vi "DSF.Shared.Configuration.Transfer.Initialize.vi"(7 "direction":T1, 8 "error in (no error)":errorcluster, 10 "Transfer Configuration cluster":T2, 11 "Transfer Configuration in":refnum<class "VeriStand DSF.Transfer.Configuration.lvclass">) -> (0 "error out":errorcluster, 3 "Transfer Configuration out":refnum<class "VeriStand DSF.Transfer.Configuration.lvclass">)   [LabVIEW 2017, in "Data Sharing Framework Engine.lvlib" / "VeriStand DSF.Transfer.Configuration.lvclass"]
uses:
  VeriStand DSF.Transfer.Configuration.lvclass
  DSF Core/Built/PharLap x86/Engine/c/DSF.Engine.lvlibp/DSF Configuration API/1.0.0/Public/Controls/DSF Engine Transfer Configuration.ctl
  DSF Core/Built/PharLap x86/Engine/c/DSF.Engine.lvlibp/DSF Configuration API/1.0.0/Public/Controls/DSF Byte Order.ctl
  DSF Core/Built/PharLap x86/Engine/c/DSF.Engine.lvlibp/DSF Configuration API/1.0.0/Public/Controls/DSF Engine Channel Configuration.ctl
  DSF Core/Built/PharLap x86/Engine/c/DSF.Engine.lvlibp/DSF Configuration API/1.0.0/Public/Controls/DSF Data Type.ctl
  DSF Core/Built/PharLap x86/Engine/c/DSF.Engine.lvlibp/DSF Configuration API/1.0.0/Public/Controls/DSF Settings Info.ctl
  DSF Core/Built/PharLap x86/Engine/c/DSF.Engine.lvlibp/DSF Configuration API/1.0.0/Public/Controls/DSF Direction.ctl
  VeriStand DSF.Transfer.Configuration.lvclass/VeriStand DSF.Transfer.Configuration.ctl
  <vilib>/NI Veristand/Custom Device API/Custom Device Channel Type.ctl
  <vilib>/NI Veristand/Custom Device API/Data Access Type.ctl
  DSF Core/Built/PharLap x86/Engine/c/DSF.Engine.lvlibp/Shared/Classes/Transfer/DSF.Shared.Configuration.Transfer.lvclass
  <vilib>/NI Veristand/Custom Device API/Custom Device API.lvlib
  DSF Core/Built/PharLap x86/Engine/c/DSF.Engine.lvlibp/DSF Configuration API/1.0.0/DSF Configuration API.lvlib
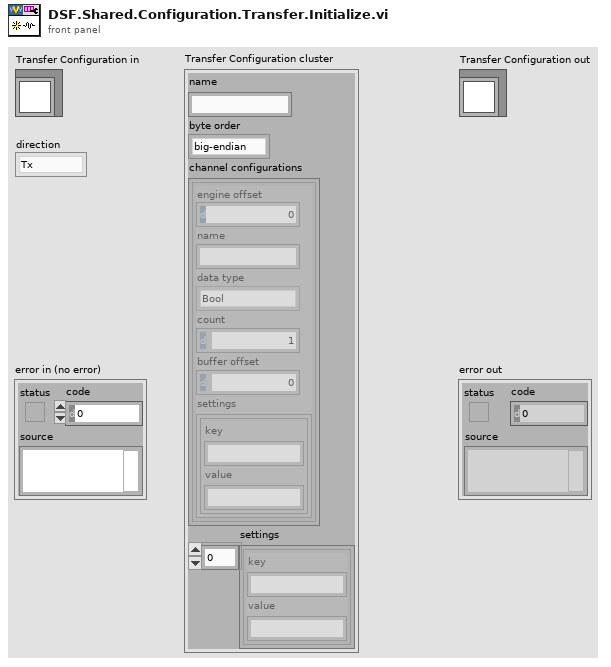
[diagram p1: front panel]
types:
  T1 = typedef "DSF.Engine.lvlibp/DSF Configuration API.lvlib/DSF Direction.ctl" = enum8{"Tx", "Rx"}
  T2 = typedef "DSF.Engine.lvlibp/DSF Configuration API.lvlib/DSF Engine Transfer Configuration.ctl" = cluster{"name":string, "byte order":T3, "channel configurations":T4[], "settings":T6}
  T3 = typedef "DSF.Engine.lvlibp/DSF Configuration API.lvlib/DSF Byte Order.ctl" = enum8{"big-endian", "little-endian"}
  T4 = typedef "DSF.Engine.lvlibp/DSF Configuration API.lvlib/DSF Engine Channel Configuration.ctl" = cluster{"engine offset":u64, "name":string, "data type":T5, "count":u64, "buffer offset":u64, "settings":T6}
  T5 = typedef "DSF.Engine.lvlibp/DSF Configuration API.lvlib/DSF Data Type.ctl" = enum8{"Bool", "SGL", "DBL", "I8", "I16", "I32", "I64", "U8", "U16", "U32", "U64"}
  T6 = typedef "DSF.Engine.lvlibp/DSF Configuration API.lvlib/DSF Settings Info.ctl" = cluster{"key":string, "value":string}[]
  T7 = typedef "Custom Device API.lvlib/Data Access Type.ctl" = enum16{"Read", "Write"}
  T8 = typedef "Custom Device API.lvlib/Custom Device Channel Type.ctl" = enum16{"Input", "Output"}
  T9 = typedef "Custom Device API.lvlib/Custom Device Item Ref.ctl" = u64
  T10 = typedef "Custom Device API.lvlib/Data Reference.ctl" = i32
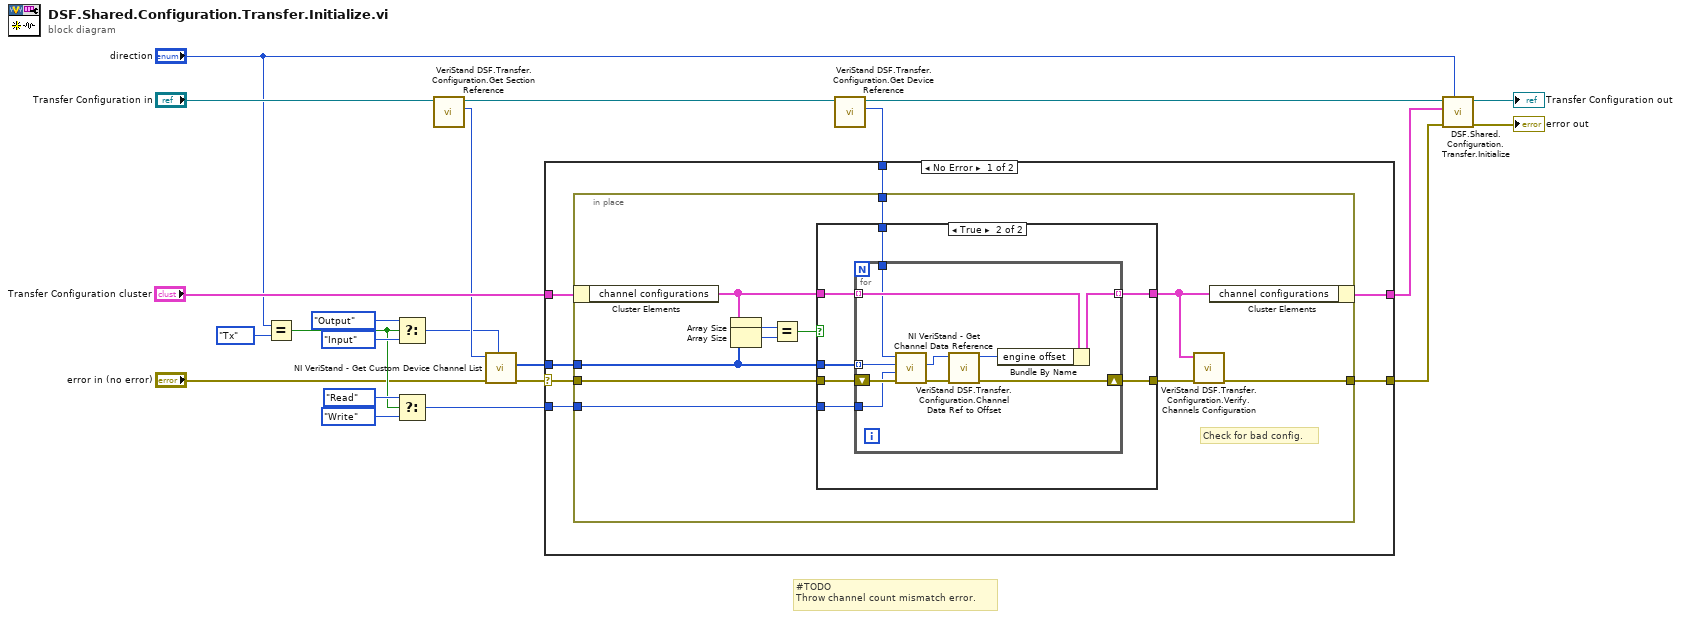
[diagram p0: block diagram]
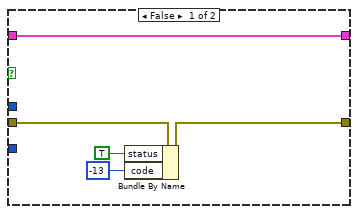
[diagram p2: hidden frame]
diagram:
  # "#TODO\nThrow channel count mismatch error."
  n1 = Equal?(x="direction", y=DSF_Direction."Tx") -> (x = y?=w15:bool)
  n2 = Select(t=Custom_Device_Channel_Type."Output" ("Channel Type"), s=w15, f=Custom_Device_Channel_Type."Input" ("Channel Type")) -> (s? t:f=w1:T8)
  n3 = Select(t=Data_Access_Type."Read" ("Access"), s=w15, f=Data_Access_Type."Write" ("Access")) -> (s? t:f=w16:T7)
  n4 = call "VeriStand DSF.Transfer.Configuration.Get Section Reference.vi"("VeriStand DSF.Transfer.Configuration in"="Transfer Configuration in") -> ("Section Ref"=w11:T9, "VeriStand DSF.Transfer.Configuration out"=w4:refnum<class "VeriStand DSF.Transfer.Configuration.lvclass">)  [unwired: 9 in]
  n5 = call <vilib>:"NI VeriStand - Get Custom Device Channel List.vi"("Channel Type"=w1, "error in (no error)"="error in (no error)", "Device Ref in"=w11) -> ("error out"=w5:errorcluster, "Specified Channel Ref List"=w6:T9[])  [unwired: 6 in, 1 out]
  n6 = call "VeriStand DSF.Transfer.Configuration.Get Device Reference.vi"("VeriStand DSF.Transfer.Configuration in"=w4) -> ("Device Reference"=w2:T9, "VeriStand DSF.Transfer.Configuration out"=w3:refnum<class "VeriStand DSF.Transfer.Configuration.lvclass">)  [unwired: 9 in]
  n7 = case shown="No Error" w5 {
    selector: w5 -> [w24 w63]
    tunnel: w16 -> [w29 _]
    tunnel: "Transfer Configuration cluster" -> [w28 _]
    tunnel: [w27 _] -> w9
    tunnel: [w26 w63] -> w7
    tunnel: w6 -> [w25 _]
    tunnel: w2 -> [w23 _]
    frame No Error {
      n8 = in-place {
        in-place-border: w24 -> [w40]
        in-place-border: w25 -> [w36]
        in-place-border: w29 -> [w38]
        in-place-border: [w34] -> w26
        in-place-border: w23 -> [w30]
        # "Check for bad config."
        n9 = in-place-cluster #1(w28) -> ("channel configurations"=w37:T4[])
        n10 = Array Size(array=w37) -> (size(s)=w32:i32)
        n11 = Array Size(array=w36) -> (size(s)=w31:i32)
        n12 = Equal?(x=w32, y=w31) -> (x = y?=w39:bool)
        n13 = case shown="True" w39 {
          tunnel: w40 -> [w45 w52]
          tunnel: [w44 w51] -> w35
          tunnel: w36 -> [_ w50]
          tunnel: w38 -> [_ w49]
          tunnel: w37 -> [w42 w48]
          tunnel: [w42 w47] -> w33
          tunnel: w30 -> [_ w46]
          frame False {
            n14 = Bundle By Name(cluster=w45, "status"=TRUE, "code"=-13) -> (w44:errorcluster)
          }
          frame True {
            n15 = for {
              tunnel: w50 -> [w61] mode=indexing
              shift-right: [w58] -> w51
              shift-left: w52 -> [w62]
              tunnel: w49 -> [w60]
              tunnel: w48 -> [w55] mode=indexing
              tunnel: [w54] -> w47 mode=indexing
              tunnel: w46 -> [w53]
              n16 = call <vilib>:"NI VeriStand - Get Channel Data Reference.vi"("error in (no error)"=w62, "Access"=w60, "Channel Ref in"=w61, "Device Ref in"=w53) -> ("error out"=w59:errorcluster, "Channel Data Reference"=w57:T10)  [unwired: 6 out]
              n17 = call "VeriStand DSF.Transfer.Configuration.Channel Data Ref to Offset.vi"("error in (no error)"=w59, "Channel Data Reference"=w57) -> ("error out"=w58:errorcluster, "channel offset"=w56:u64)  [unwired: 8 in]
              n18 = Bundle By Name(cluster=w55, "engine offset"=w56) -> (w54:T4)
            }
          }
        }
        n19 = call "VeriStand DSF.Transfer.Configuration.Verify.Channels Configuration.vi"("error in (no error)"=w35, "channel configurations"=w33) -> ("error out"=w34:errorcluster)  [unwired: 9 in]
        n20 = in-place-cluster #1("channel configurations"=w33) -> (w27:T2)
      }
    }
    frame Error {
    }
  }
  n21 = call-parent "DSF.Shared.Configuration.Transfer.Initialize.vi"("direction"="direction", "error in (no error)"=w7, "Transfer Configuration cluster"=w9, "Transfer Configuration in"=w3) -> ("error out"=→"error out":errorcluster, "Transfer Configuration out"=→"Transfer Configuration out":refnum<class "VeriStand DSF.Transfer.Configuration.lvclass">)  [unwired: 6 in]
